vi "Test XTrend.vi"() -> ()   [LabVIEW 2015]
uses:
  XTrend.xctl
  View Mode.ctl
panel:
  out "XTrend":dbl[](xcontrol)
  in  "View Mode":T1
  in  "Trending Threshold":dbl=100.0
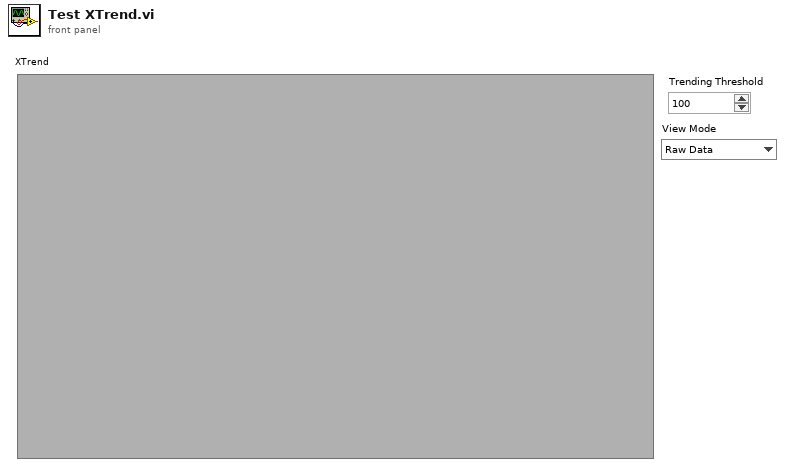
[diagram p1: front panel]
types:
  T1 = typedef "View Mode.ctl" = enum16{"Raw Data", "Trend"}
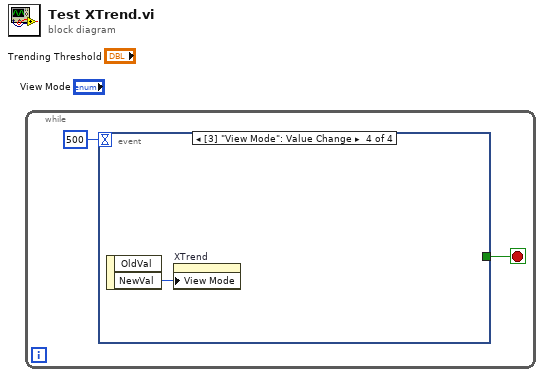
[diagram p0: block diagram]
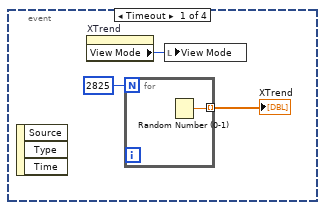
[diagram p2: hidden frame]
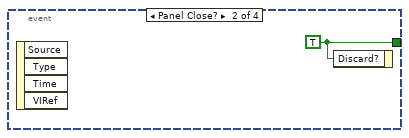
[diagram p3: hidden frame]
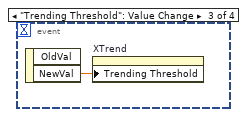
[diagram p4: hidden frame]
diagram:
  n1 = while {
    stop <- w1 stop-if-true
    n2 = event shown="[3] \"View Mode\": Value Change" {
      selector: _ -> [_ _ _ _]
      dyn-events: _ -> [_ _ _ _]
      timeout: 500 -> [_ _ _ _]
      tunnel: [_ w7 _ _] -> w1
      event Timeout {
        n3 = event-data() -> ()  [unwired: 1 in, 3 out]
        n4 = property on="XTrend" class="XTrend (strict)"() -> ("View Mode"=w3:T1)  [unwired: 2 in, 2 out]
        n5 = for {
          N: 2825 -> [_]
          tunnel: [w6] -> w5 mode=indexing
          n6 = Random Number (0-1)() -> (number: 0 to 1=w6:dbl)
        }
        "XTrend" <- w5
        n7 = local write "View Mode"(w3) -> ()
      }
      event Panel Close? {
        w7 = TRUE ("Discard?")
        n8 = event-data() -> ()  [unwired: 1 in, 4 out]
        n9 = event-data("Discard?"=w7) -> ()  [unwired: 1 in, 1 out]
      }
      event "Trending Threshold": Value Change {
        n10 = event-data() -> ("NewVal"=w8:dbl)  [unwired: 1 in, 1 out]
        n11 = property on="XTrend" class="XTrend (strict)"("Trending Threshold"=w8) -> ()  [unwired: 2 in, 2 out]
      }
      event Value Change {
        n12 = event-data() -> ("NewVal"=w9:T1)  [unwired: 1 in, 1 out]
        n13 = property on="XTrend" class="XTrend (strict)"("View Mode"=w9) -> ()  [unwired: 2 in, 2 out]
      }
    }
  }
